vi "Count Down by One.vi"(8 "error in (no error)":errorcluster, 11 "Worker in":refnum<class "Worker.lvclass">) -> (0 "error out":errorcluster, 3 "Worker out":refnum<class "Worker.lvclass">)   [LabVIEW 2024, in "Worker.lvlib" / "Worker.lvclass"]
uses:
  Worker.lvclass
  Worker.lvclass/Worker.ctl
  <vilib>/ActorFramework/Actor/Actor.lvclass
  Chef State Logic/Work Logic Messages/Update Count Msg/Update Count Msg.lvclass
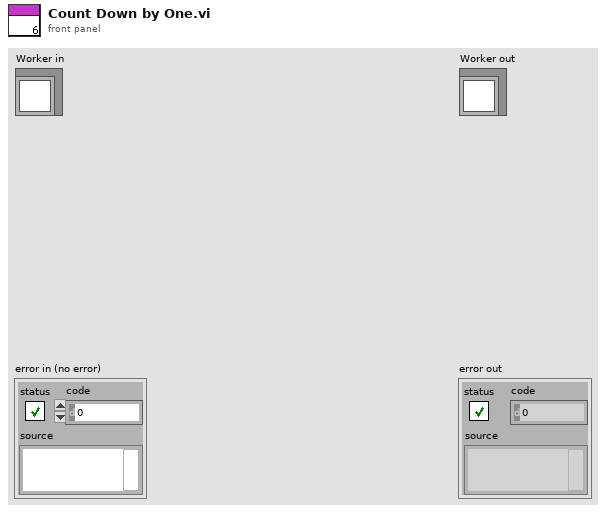
[diagram p1: front panel]
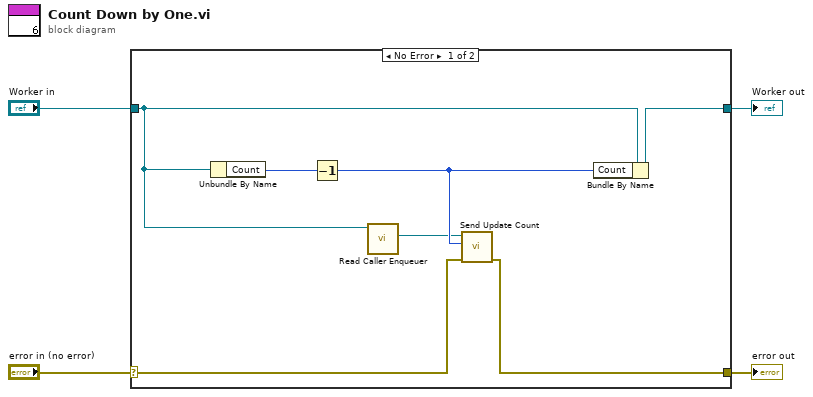
[diagram p0: block diagram]
diagram:
  n1 = case shown="No Error" "error in (no error)" {
    selector: "error in (no error)" -> [w8 w13]
    tunnel: [w7 w13] -> w3
    tunnel: [w10 w12] -> w1
    tunnel: "Worker in" -> [w9 w12]
    frame No Error {
      n2 = Unbundle By Name(w9) -> ("Count"=w11:u64)
      n3 = Decrement(x=w11) -> (x-1=w6:u64)
      n4 = call <vilib>:"Read Caller Enqueuer.vi"("Actor"=w9) -> ("Caller Enqueuer"=w5:refnum<class "Message Enqueuer.lvclass">)  [unwired: 10 in]
      n5 = call "Send Update Count.vi"("error in (no error)"=w8, "Numeric"=w6, "Message Enqueuer"=w5) -> ("error out"=w7:errorcluster)  [unwired: 7 in, 1 out]
      n6 = Bundle By Name(cluster=w9, "Count"=w6) -> (w10:refnum<class "Worker.lvclass">)
    }
    frame Error {
    }
  }
  "error out" <- w3
  "Worker out" <- w1
